vi "Set Thread ID Pool.vi"(10 "Thread ID Pool":refnum<class "Pool ID.lvclass">, 11 "Plugin in":refnum<class "Plugin.lvclass">) -> (3 "Plugin out":refnum<class "Plugin.lvclass">)   [LabVIEW 2017, in "Data Sharing Framework Core.lvlib" / "Data Sharing Framework Engine.lvlib" / "Plugin.lvclass"]
uses:
  Plugin.lvclass
  Internal/Execution/Pool/Pool ID/Pool ID.lvclass
  Plugin.lvclass/Plugin.ctl
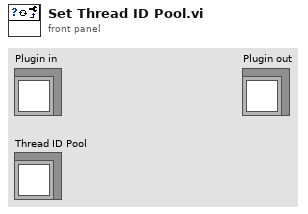
[diagram p1: front panel]
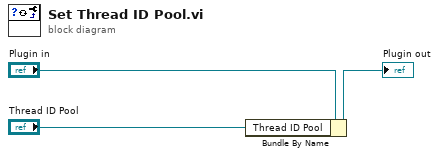
[diagram p0: block diagram]
diagram:
  n1 = Bundle By Name(cluster="Plugin in", "Thread ID Pool"="Thread ID Pool") -> (→"Plugin out":refnum<class "Plugin.lvclass">)
